vi "QueryExcuseContent.vi"(8 "error in (no error)":errorcluster, 9 "Name":string, 10 "TableName":string, 11 "ExcuseNotesHandler":refnum<class "ExcuseNotesHandler.lvclass">) -> (0 "error out":errorcluster, 2 "ExcuseNote(\"\")":string[][](array[string]), 3 "ExcuseNotesHandler Out":refnum<class "ExcuseNotesHandler.lvclass">)   [LabVIEW 2015, in "Admin_Actor.lvlib" / "ExcuseNotesHandler.lvclass"]
uses:
  ExcuseNotesHandler.lvclass
  ExcuseNotesHandler.lvclass/ExcuseNotesHandler.ctl
  API/_Database/Database.lvclass
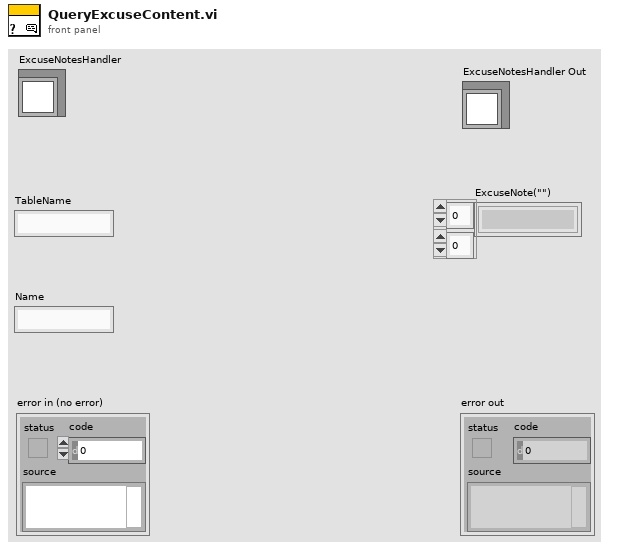
[diagram p1: front panel]
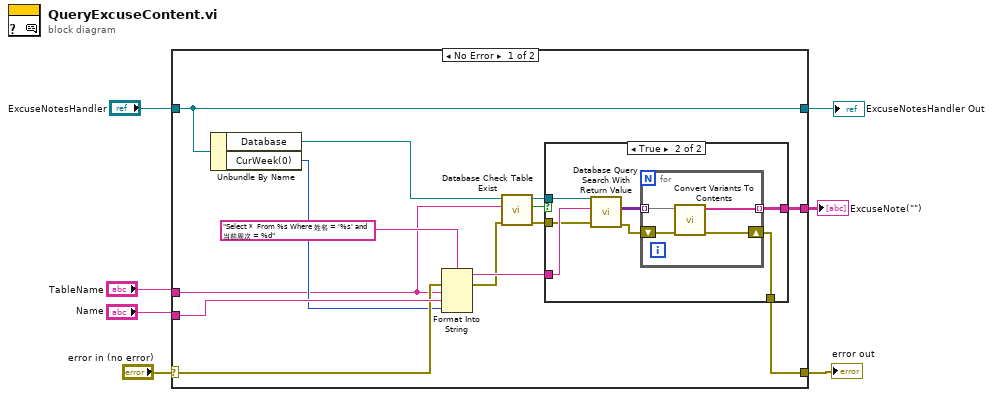
[diagram p0: block diagram]
diagram:
  n1 = case shown="No Error" "error in (no error)" {
    selector: "error in (no error)" -> [w19 w35]
    tunnel: [w17 w35] -> w6
    tunnel: [w21 w34] -> w1
    tunnel: "ExcuseNotesHandler" -> [w21 w34]
    tunnel: "TableName" -> [w13 _]
    tunnel: "Name" -> [w20 _]
    tunnel: [w16 _] -> w3
    frame No Error {
      n2 = Unbundle By Name(w21) -> ("Database"=w12:refnum<class "Database.lvclass">, "CurWeek(0)"=w15:i32)
      n3 = Format Into String(format string="Select *  From %s Where 姓名 = '%s' and 当前周次 = %d" ("SQL query"), error in=w19, w13, w20, w15) -> (resulting string=w18:string, error out=w11:errorcluster)  [unwired: 1 in]
      n4 = call "Database Check Table Exist.vi"("error in (no error)"=w11, "Table"=w13, "Database in"=w12) -> ("error out"=w9:errorcluster, "Exit?"=w10:bool, "Database out"=w8:refnum<class "Database.lvclass">)  [unwired: 6 in]
      n5 = case shown="True" w10 {
        tunnel: w18 -> [_ w28]
        tunnel: [w22 w26] -> w17
        tunnel: [_ w25] -> w16
        tunnel: w9 -> [w22 w24]
        tunnel: w8 -> [_ w23]
        frame False {
        }
        frame True {
          n6 = call "Database Query Search With Return Value.vi"("error in (no error)"=w24, "SQL query"=w28, "object in"=w23) -> ("error out"=w27:errorcluster, "recordset data"=w29:variant[][])  [unwired: 5 in, 2 out]
          n7 = for {
            tunnel: w29 -> [w33] mode=indexing
            tunnel: [w31] -> w25 mode=indexing
            shift-right: [w30] -> w26
            shift-left: w27 -> [w32]
            n8 = call "Convert Variants To Contents.vi"("error in"=w32, "ExcuseNote"=w33) -> ("error out"=w30:errorcluster, "ExcuseNote(\"\")"=w31:string[])  [unwired: 8 in]
          }
        }
      }
    }
    frame Error {
    }
  }
  "error out" <- w6
  "ExcuseNote(\"\")" <- w3
  "ExcuseNotesHandler Out" <- w1
